vi "Teleop.vi"(10 "Match Info":T1={"Autonomous Elapsed Seconds"=0.0, "TeleOp Elapsed Seconds"=0.0, "Disabled Elapsed Seconds"=0.0, "Visited Autonomous"=FALSE, "Visited TeleOp"=FALSE, "Visited Disabled"=FALSE, "Autonomous Settings"={"Autonomous Style"=enum."Independent", "VI Refnum"=refnum}}, 11 "Call Context":T2) -> ()   [LabVIEW 2018]
doc: "This VI is called for each enabled TeleOp packet received from the DS. It is typically used to read from joysticks and other inputs and update I/O or setpoints for timed control loops. It should complete and return within 20 milliseconds or risk missing DS packets."
uses:
  <vilib>/Rock Robotics/WPI/DriverStation/WPI_DriverStationDerivedRobotMode.ctl
  <vilib>/Rock Robotics/WPI/DriverStation/WPI_DriverStationMatch Info.ctl
  <vilib>/Rock Robotics/WPI/Utilities/WPI_GetSetVariantRefNum.vi
  <vilib>/Rock Robotics/Network Tables/NT Write Boolean Array.vi
  <vilib>/Rock Robotics/Network Tables/NT Write Numeric Array.vi
  <vilib>/Rock Robotics/Network Tables/NT Read Number.vi
  Framework/Robot Global Data.vi
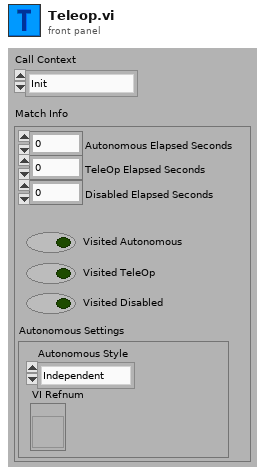
[diagram p1: front panel]
types:
  T1 = typedef "WPI_DriverStationMatch Info.ctl" = cluster{"Autonomous Elapsed Seconds":dbl, "TeleOp Elapsed Seconds":dbl, "Disabled Elapsed Seconds":dbl, "Visited Autonomous":bool, "Visited TeleOp":bool, "Visited Disabled":bool, "Autonomous Settings":cluster{"Autonomous Style":enum16{"Iterative", "Independent"}, "VI Refnum":refnum<vi>}}
  T2 = typedef "WPI_DriverStationDerivedRobotMode.ctl" = enum16{"Init", "Execute", "Stop"}
  T3 = typedef "WPI_JoystickDevRef.ctl" = cluster{"Device":T4}
  T4 = typedef "WPI_JoystickDeviceEnum.ctl" = enum16{"USB 0", "USB 1", "USB 2", "USB 3", "USB 4", "USB 5"}
  T5 = typedef "Command Status Info.ctl" = cluster{"Name":string, "Status":T6, "notifier out":T7}
  T6 = typedef "Completion Status.ctl" = enum16{"Successful", "Aborted", "Incomplete"}
  T7 = typedef "Completion Notifier.ctl" = refnum<notifier>
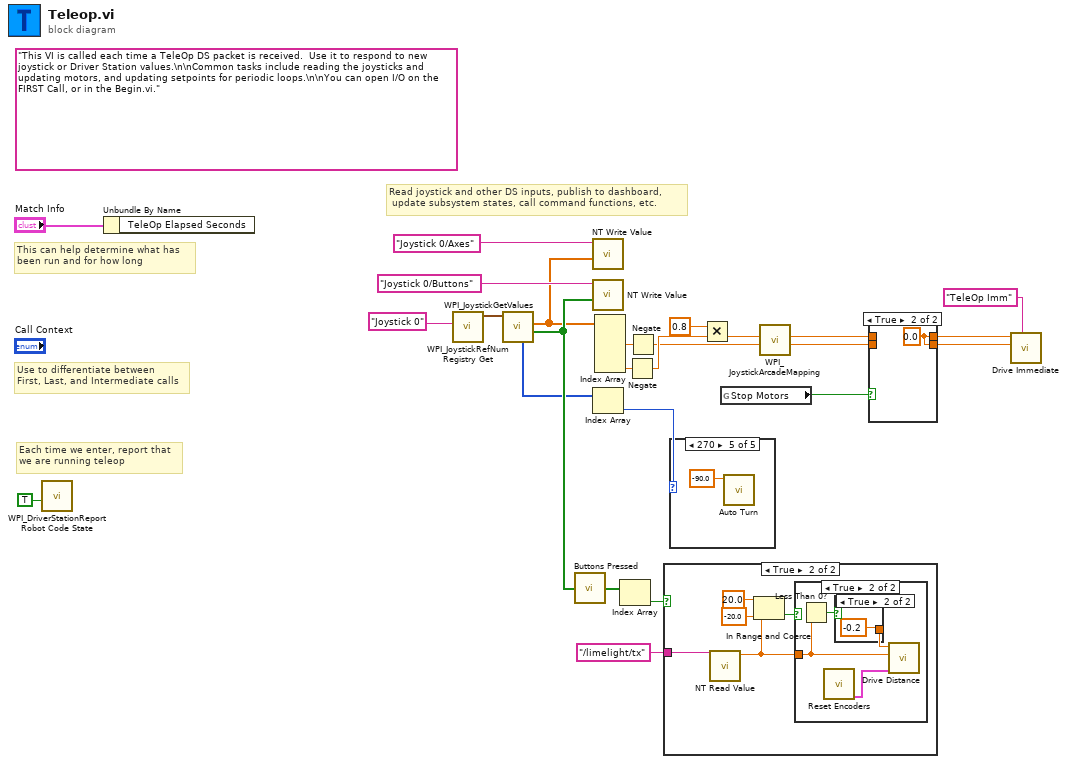
[diagram p0: block diagram]
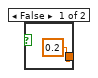
[diagram p4: hidden frame]
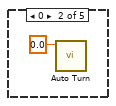
[diagram p6: hidden frame]
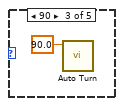
[diagram p7: hidden frame]
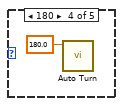
[diagram p8: hidden frame]
diagram:
  (unwired) "This VI is called each time a TeleOp DS packet is received.  Use it to respond to new joystick or Driver Station values.\n\nCommon tasks include reading the joysticks and updating motors, and updating setpoints for periodic loops.\n\nYou can open I/O on the FIRST Call, or in the Begin.vi."
  # "Read joystick and other DS inputs, publish to dashboard,\n update subsystem states, call command functions, etc."
  # "Each time we enter, report that\nwe are running teleop"
  # "Use to differentiate between\nFirst, Last, and Intermediate calls"
  # "This can help determine what has\nbeen run and for how long"
  n1 = call <vilib>:"WPI_DriverStationReport Robot Code State.vi"("TeleOp"=TRUE ("Autonomous")) -> ()  [unwired: 10 in, 1 out]
  n2 = Unbundle By Name("Match Info") -> ()  [unwired: 1 out]
  n3 = call <vilib>:"WPI_JoystickRefNum Registry Get.vi"("refnum name"="Joystick 0") -> ("JoystickDevRef"=w22:T3)  [unwired: 1 in, 9 out]
  n4 = call <vilib>:"WPI_JoystickGetValues.vi"("JoystickDevRef"=w22) -> ("Buttons"=w18:bool[], "Axes"=w17:dbl[], "POVs"=w5:i16[])  [unwired: 6 in, 2 out]
  n5 = call "Buttons Pressed.vi"("Button Values"=w18) -> ("Button Presses"=w3:bool[])
  n6 = call-poly <vilib>:"NT Write Value.vi"("Numeric Array"=w17, "Name"="Joystick 0/Axes") -> ()  [unwired: 9 in, 1 out]
  n7 = call-poly <vilib>:"NT Write Value.vi"("Boolean Array"=w18, "Name"="Joystick 0/Buttons") -> ()  [unwired: 9 in, 1 out]
  n8 = Index Array(array=w5) -> (element=w4:i16)  [unwired: 1 in]
  n9 = Index Array(array=w17) -> (element #2=w20:dbl, element #5=w11:dbl)  [unwired: 5 in, 3 out]
  n10 = Index Array(array=w3) -> (element=w2:bool)  [unwired: 1 in]
  n11 = Negate(x=w11) -> (-x=w15:dbl)
  n12 = Negate(x=w20) -> (-x=w14:dbl)
  n13 = case shown="True" w2 {
    tunnel: "/limelight/tx" ("Name") -> [_ w30]
    frame False {
    }
    frame True {
      n14 = call-poly <vilib>:"NT Read Value.vi"("Name"=w30) -> ("Numeric"=w27:dbl)  [unwired: 9 in, 1 out]
      n15 = In Range and Coerce(upper limit=20.0, x=w27, lower limit=-20.0) -> (In Range?=w26:bool)  [unwired: 1 out]
      n16 = case shown="True" w26 {
        tunnel: w27 -> [_ w32]
        frame False {
        }
        frame True {
          n17 = Less Than 0?(x=w32) -> (x < 0?=w33:bool)
          n18 = call "Reset Encoders.vi"() -> ("Command Info Out"=w31:T5)  [unwired: 11 in]
          n19 = case shown="True" w33 {
            tunnel: [0.2 ("Speed") -0.2 ("Speed")] -> w34
            frame False {
            }
            frame True {
            }
          }
          n20 = call "Drive Distance.vi"("Command Info In"=w31, "Distance"=w32, "Speed"=w34) -> ()  [unwired: 8 in, 1 out]
        }
      }
    }
  }
  n21 = case shown="270" w4 {
    frame -1, Default {
    }
    frame 0 {
      n22 = call "Auto Turn.vi"("Target Angle"=0.0) -> ()  [unwired: 10 in, 1 out]
    }
    frame 90 {
      n23 = call "Auto Turn.vi"("Target Angle"=90.0) -> ()  [unwired: 10 in, 1 out]
    }
    frame 180 {
      n24 = call "Auto Turn.vi"("Target Angle"=180.0) -> ()  [unwired: 10 in, 1 out]
    }
    frame 270 {
      n25 = call "Auto Turn.vi"("Target Angle"=-90.0) -> ()  [unwired: 10 in, 1 out]
    }
  }
  n26 = Multiply(x=0.8, y=w15) -> (x*y=w13:dbl)
  n27 = global read "Robot Global Data.vi" "Stop Motors"() -> (w10:bool)
  n28 = call <vilib>:"WPI_JoystickArcadeMapping.vi"("Y axis value"=w14, "X axis value"=w13) -> ("Right Motor Value"=w8:dbl, "Left Motor Value"=w9:dbl)  [unwired: 8 in]
  n29 = case shown="True" w10 {
    tunnel: w9 -> [w42 _]
    tunnel: w8 -> [w41 _]
    tunnel: [w42 w43] -> w7
    tunnel: [w41 w43] -> w6
    frame False {
    }
    frame True {
      w43 = 0.0 ("Left Motor Value")
    }
  }
  n30 = call "Drive Immediate.vi"("Description"="TeleOp Imm", "Right Setpoint"=w6, "Left Setpoint"=w7) -> ()  [unwired: 8 in, 1 out]
